vi "Table verify colomn.vi"(0 "PDF Report":refnum<class "PDF Report Class.lvclass">, 5 "numColumns":i32, 9 "columnWidth":sgl[](array[numeric]), 11 "error in (no error)":errorcluster, 12 "Pages dimensions":T1={"Start at page"=-1, "Page Size"=0, "Orientation"=enum."Landscape", "widht"=792.0, "height"=72.0, "Margin left"=72.0, "Margin right"=72.0, "Margin top"=72.0, "Margin bottom"=72.0, "X0"=0.0, "X1"=612.0, "Y0"=0.0, "Y1"=792.0} {"Page Size" items=["Custom", "LETTER", "NOTE", "LEGAL", "TABLOID", "EXECUTIVE", "POSTCARD", "A0", "A1", "A2", "A3", "A4", "A5", "A6", "A7", "A8", "A9", "A10", "B0", "B1", "B2", "B3", "B4", "B5", "B6", "B7", "B8", "B9", "B10", "ARCH_E", "ARCH_D", "ARCH_C", "ARCH_B", "ARCH_A", "FLSA", "FLSE", "HALFLETTER", "_11X17", "ID_1", "ID_2", "ID_3", "LEDGER", "CROWN_QUARTO", "LARGE_CROWN_QUARTO", "DEMY_QUARTO", "ROYAL_QUARTO", "CROWN_OCTAVO", "LARGE_CROWN_OCTAVO", "DEMY_OCTAVO", "ROYAL_OCTAVO", "SMALL_PAPERBACK", "PENGUIN_SMALL_PAPERBACK", "PENGUIN_LARGE_PAPERBACK"]}) -> (4 "PDF Report duplicate":refnum<class "PDF Report Class.lvclass">, 6 "numColumns duplicate":i32, 10 "columnWidth (points)":sgl[](array[numeric]), 15 "error out":errorcluster)   [LabVIEW 2019, in "Exaprom PDF.lvlib"]
doc: "Version 1.0\nDeveloped by Jean-Marc Simard\nCopyright © 2010, Exaprom Inc.\nAll rights reserved.\nLicense: BSD\n\nWith iTextSharp 4.1.6 (http://itextsharp.sourceforge.net)\nunder Mozilla Public License Version 1.1\n(http://www.mozilla.org/MPL/MPL-1.1.html)"
uses:
  LV Class/PDF Report Class/PDF Report Class.lvclass
  Controls/Page Controls/Page dimensions.ctl
  Controls/Page Controls/Page size.ctl
  Controls/Page Controls/Page Orientation.ctl
  Controls/Initialization Controls/Unit.ctl
  Exaprom PDF.lvlib
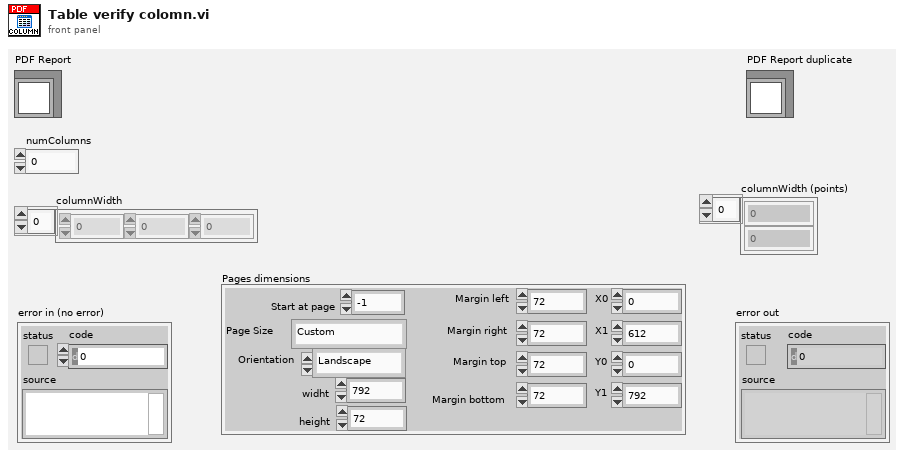
[diagram p1: front panel]
types:
  T1 = typedef "Exaprom PDF.lvlib/Page dimensions.ctl" = cluster{"Start at page":i32, "Page Size":T2, "Orientation":T3, "widht":sgl, "height":sgl, "Margin left":sgl, "Margin right":sgl, "Margin top":sgl, "Margin bottom":sgl, "X0":sgl, "X1":sgl, "Y0":sgl, "Y1":sgl}
  T2 = typedef "Exaprom PDF.lvlib/Page size.ctl" = i32
  T3 = typedef "Exaprom PDF.lvlib/Page Orientation.ctl" = enum16{"Portrait", "Landscape"}
  T4 = typedef "Exaprom PDF.lvlib/Unit.ctl" = enum16{"inch", "mm"}
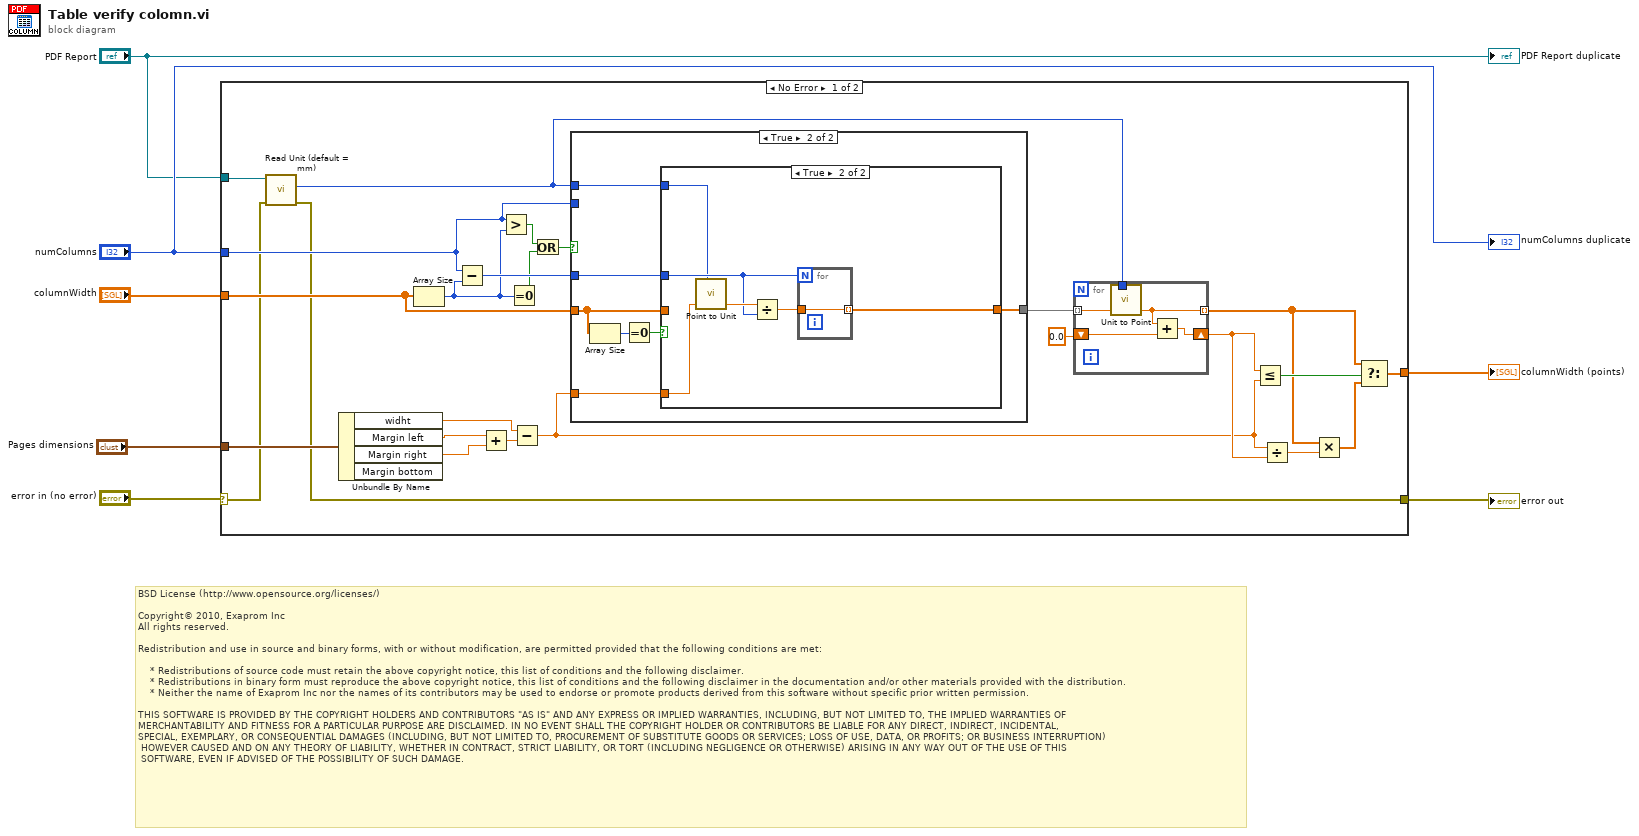
[diagram p0: block diagram]
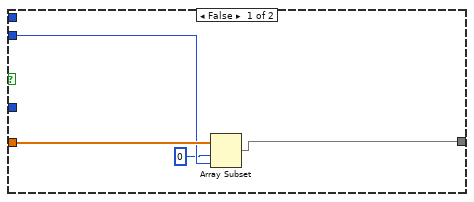
[diagram p2: hidden frame]
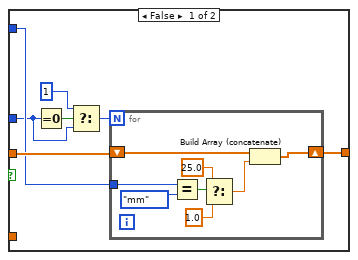
[diagram p3: hidden frame]
diagram:
  # "BSD License (http://www.opensource.org/licenses/)\n\nCopyright© 2010, Exaprom Inc\nAll rights reserved.\n\nRedistribution and use in source and binary forms, with or without modification, are permitted provided that the following conditions are met:\n\n    * Redistributions of source code must retain the above copyright notice, this list of conditions and the following disclaimer.\n    * Redistributions in binary form must reproduce the above copyright notice, this list of conditions and the following disclaimer in the documentation and/or other materials provided with the distribution.\n    * Neither the name of Exaprom Inc nor the names of its contributors may be used to endorse or promote products derived from this software without specific prior written permission.\n\nTHIS SOFTWARE IS PROVIDED BY THE COPYRIGHT HOLDERS AND CONTRIBUTORS \"AS IS\" AND ANY EXPRESS OR IMPLIED WARRANTIES, INCLUDING, BUT NOT LIMITED TO, THE IMPLIED WARRANTIES OF \nMERCHANTABILITY AND FITNESS FOR A PARTICULAR PURPOSE ARE DISCLAIMED. IN NO EVENT SHALL THE COPYRIGHT HOLDER OR CONTRIBUTORS BE LIABLE FOR ANY DIRECT, INDIRECT, INCIDENTAL,\nSPECIAL, EXEMPLARY, OR CONSEQUENTIAL DAMAGES (INCLUDING, BUT NOT LIMITED TO, PROCUREMENT OF SUBSTITUTE GOODS OR SERVICES; LOSS OF USE, DATA, OR PROFITS; OR BUSINESS INTERRUPTION)\n HOWEVER CAUSED AND ON ANY THEORY OF LIABILITY, WHETHER IN CONTRACT, STRICT LIABILITY, OR TORT (INCLUDING NEGLIGENCE OR OTHERWISE) ARISING IN ANY WAY OUT OF THE USE OF THIS\n SOFTWARE, EVEN IF ADVISED OF THE POSSIBILITY OF SUCH DAMAGE."
  n1 = case shown="No Error" "error in (no error)" {
    selector: "error in (no error)" -> [w9 w72]
    tunnel: "columnWidth" -> [w17 w71]
    tunnel: "numColumns" -> [w23 _]
    tunnel: "Pages dimensions" -> [w18 _]
    tunnel: [w19 w71] -> w6
    tunnel: [w8 w72] -> w4
    tunnel: "PDF Report" -> [w15 _]
    frame No Error {
      n2 = call-dynamic "Read Unit (default = mm).vi"("error in (no error)"=w9, "PDF Report Class in"=w15) -> ("error out"=w8:errorcluster, "Unit (default = mm)"=w10:T4)  [unwired: 7 in, 1 out]
      n3 = Unbundle By Name(w18) -> ("widht"=w31:sgl, "Margin left"=w29:sgl, "Margin right"=w30:sgl)  [unwired: 1 out]
      n4 = Array Size(array=w17) -> (size(s)=w11:i32)
      n5 = Subtract(x=w23, y=w11) -> (x-y=w24:i32)
      n6 = Add(x=w29, y=w30) -> (x+y=w32:sgl)
      n7 = Greater?(x=w23, y=w11) -> (0:w13:bool)
      n8 = Equal To 0?(x=w11) -> (x = 0?=w12:bool)
      n9 = Subtract(x=w31, y=w32) -> (x-y=w16:sgl)
      n10 = Or(x=w13, y=w12) -> (x .or. y?=w14:bool)
      n11 = case shown="True" w14 {
        tunnel: w17 -> [w36 w41]
        tunnel: w24 -> [_ w43]
        tunnel: w23 -> [w35 _]
        tunnel: [w33 w42] -> w22
        tunnel: w16 -> [_ w38]
        tunnel: w10 -> [_ w37]
        frame False {
          n12 = Array Subset(array=w36, index=0, length=w35) -> (w33:sgl[])
        }
        frame True {
          n13 = Array Size(array=w41) -> (size(s)=w40:i32)
          n14 = Equal To 0?(x=w40) -> (x = 0?=w39:bool)
          n15 = case shown="True" w39 {
            tunnel: w43 -> [w45 w61]
            tunnel: [w50 w64] -> w42
            tunnel: w41 -> [w49 _]
            tunnel: w38 -> [_ w63]
            tunnel: w37 -> [w48 w59]
            frame False {
              n16 = Equal To 0?(x=w45) -> (x = 0?=w47:bool)
              n17 = Select(t=1, s=w47, f=w45) -> (s? t:f=w46:i32)
              n18 = for {
                N: w46 -> [_]
                shift-right: [w57] -> w50
                shift-left: w49 -> [w58]
                tunnel: w48 -> [w56]
                n19 = Equal?(x=w56, y=Unit."mm") -> (x = y?=w54:bool)
                n20 = Select(t=sgl 25.0 ("mm"), s=w54, f=sgl 1.0 ("mm")) -> (s? t:f=w52:sgl)
                n21 = Build Array (concatenate)(w58, w52) -> (w57:sgl[])
              }
            }
            frame True {
              n22 = call "Point to Unit.vi"("X point"=w63, "Unit (default = mm)"=w59) -> ("X unit"=w62:sgl)  [unwired: 7 out]
              n23 = Divide(x=w62, y=w61) -> (x/y=w60:sgl)
              n24 = for {
                N: w61 -> [_]
                tunnel: [w65] -> w64 mode=indexing
                tunnel: w60 -> [w65]
              }
            }
          }
        }
      }
      n25 = for {
        tunnel: w22 -> [w70] mode=indexing
        tunnel: [w68] -> w20 mode=indexing
        shift-right: [w67] -> w25
        shift-left: sgl 0.0 ("WidthPercentage") -> [w69]
        tunnel: w10 -> [w66]
        n26 = call "Unit to Point.vi"("X unit"=w70, "Unit (default = mm)"=w66) -> ("X point"=w68:sgl)  [unwired: 7 out]
        n27 = Add(x=w68, y=w69) -> (x+y=w67:sgl)
      }
      n28 = Less Or Equal?(x=w25, y=w16) -> (x <= y?=w21:bool)
      n29 = Divide(x=w16, y=w25) -> (x/y=w27:sgl)
      n30 = Multiply(x=w20, y=w27) -> (x*y=w26:sgl[])
      n31 = Select(t=w20, s=w21, f=w26) -> (s? t:f=w19:sgl[])
    }
    frame Error {
    }
  }
  "columnWidth (points)" <- w6
  "error out" <- w4
  "PDF Report duplicate" <- "PDF Report"
  "numColumns duplicate" <- "numColumns"
